vi "Count Tree Row.vi"(10 "Tree":u8, 11 "Tree Row":u8[](array[numeric])) -> (3 "Count":i64)   [LabVIEW 2021]
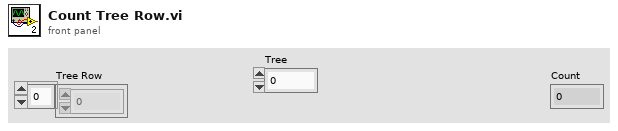
[diagram p1: front panel]
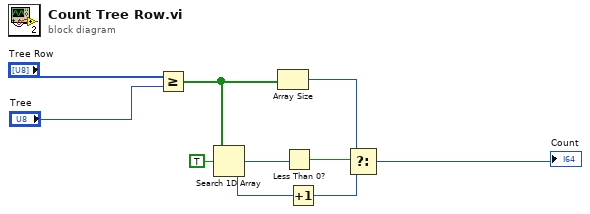
[diagram p0: block diagram]
diagram:
  n1 = Greater Or Equal?(x="Tree Row", y="Tree") -> (x >= y?=w4:bool[])
  n2 = Search 1D Array(1D array=w4, element=TRUE) -> (index of element=w2:i32)  [unwired: 1 in]
  n3 = Array Size(array=w4) -> (size(s)=w3:i32)
  n4 = Less Than 0?(x=w2) -> (x < 0?=w5:bool)
  n5 = Increment(x=w2) -> (x+1=w1:i32)
  n6 = Select(t=w3, s=w5, f=w1) -> (s? t:f=→"Count":i32)
